vi "MaterialConvert.vi"(8 "Colors Cluster":T1 {"Material"."Shine" format="%.2f"}, 9 "Array":i32[](array[numeric]), 10 "Scene.Geometry.New Mesh":refnum<vi>, 11 "Scene.New Object":refnum<vi>) -> (2 "Scene.New Object 2":refnum<vi>, 3 "Scene.Geometry.New Mesh 2":refnum<vi>)   [LabVIEW 2020, in "NI_3D Picture Control.lvlib"]
uses:
  <vilib>/picture/3D Picture Control/NI_3D Picture Control.lvlib
  <vilib>/picture/3D Picture Control/Old 3D Toolkit.llb/SkinCluster.ctl
  <vilib>/picture/3D Picture Control/Old 3D Toolkit.llb/SkinType.ctl
  <vilib>/picture/3D Picture Control/Old 3D Toolkit.llb/Material.ctl
  <vilib>/picture/3D Picture Control/NI_Old 3D Toolkit.lvlib
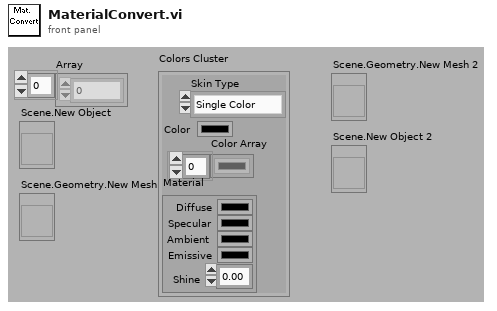
[diagram p1: front panel]
types:
  T1 = typedef "NI_3D Picture Control.lvlib/NI_Old 3D Toolkit.lvlib/SkinCluster.ctl" = cluster{"Skin Type":T2, "Color":u32, "Color Array":u32[], "Material":T3}
  T2 = typedef "NI_3D Picture Control.lvlib/NI_Old 3D Toolkit.lvlib/SkinType.ctl" = enum16{"Single Color", "Color per Vertex", "Material"}
  T3 = typedef "NI_3D Picture Control.lvlib/NI_Old 3D Toolkit.lvlib/Material.ctl" = cluster{"Diffuse":u32, "Specular":u32, "Ambient":u32, "Emissive":u32, "Shine":sgl}
  T4 = enum16{"Overall", "Per Primitive", "Per Vertex", "Binding Off"}
  T5 = enum16{"Inherit Material", "Use entire Material", "Ignore Ambient", "Ignore Diffuse", "Ignore Specular", "Ignore Emission", "Ignore Ambient and Diffuse"}
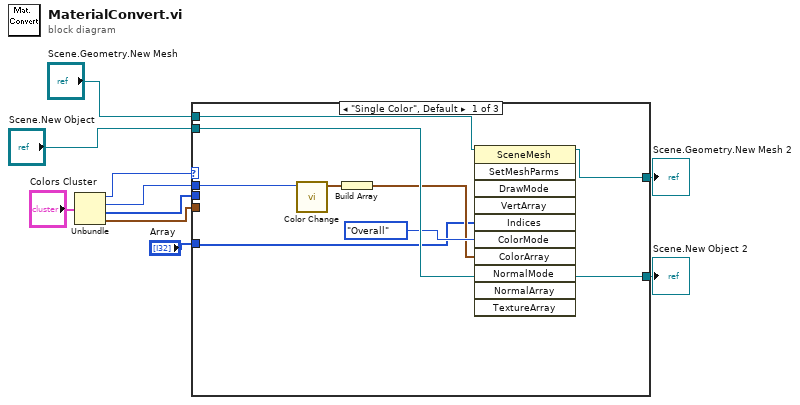
[diagram p0: block diagram]
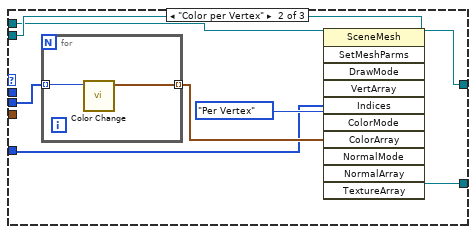
[diagram p2: hidden frame]
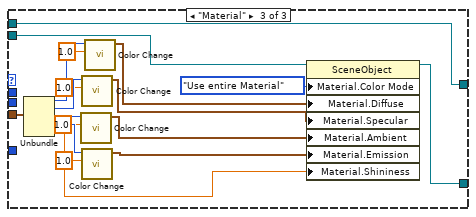
[diagram p3: hidden frame]
diagram:
  n1 = Unbundle("Colors Cluster") -> ("Skin Type"=w10:T2, "Color"=w7:u32, "Color Array"=w9:u32[], "Material"=w8:T3)
  n2 = case shown="\"Single Color\", Default" w10 {
    tunnel: w9 -> [_ w25 _]
    tunnel: w8 -> [_ _ w45]
    tunnel: "Scene.New Object" -> [w18 w24 w44]
    tunnel: w7 -> [w14 _ _]
    tunnel: [w18 w24 w39] -> w2
    tunnel: "Scene.Geometry.New Mesh" -> [w17 w23 w38]
    tunnel: "Array" -> [w11 w19 _]
    tunnel: [w16 w22 w38] -> w3
    frame "Single Color", Default {
      n3 = call <vilib>:"Color Change.vi"("Color"=w14) -> ("RGBA"=w13:cluster{"R":sgl, "G":sgl, "B":sgl, "A":sgl})  [unwired: 10 in]
      n4 = Build Array(w13) -> (w12:cluster{"R":sgl, "G":sgl, "B":sgl, "A":sgl}[])
      n5 = invoke class="SceneMesh" method="SetMeshParms"(reference=w17, "Indices"=w11, "ColorMode"=T4."Overall" ("Color Binding Mode"), "ColorArray"=w12) -> (reference out=w16:refnum<vi>)  [unwired: 7 in, 10 out]
    }
    frame "Color per Vertex" {
      n6 = for {
        tunnel: [w26] -> w20 mode=indexing
        tunnel: w25 -> [w27] mode=indexing
        n7 = call <vilib>:"Color Change.vi"("Color"=w27) -> ("RGBA"=w26:cluster{"R":sgl, "G":sgl, "B":sgl, "A":sgl})  [unwired: 10 in]
      }
      n8 = invoke class="SceneMesh" method="SetMeshParms"(reference=w23, "Indices"=w19, "ColorMode"=enum16{"Overall", "Per Primitive", "Per Vertex"}."Per Vertex" ("Color Binding Mode"), "ColorArray"=w20) -> (reference out=w22:refnum<vi>)  [unwired: 7 in, 10 out]
    }
    frame "Material" {
      n9 = Unbundle(w45) -> ("Diffuse"=w43:u32, "Specular"=w42:u32, "Ambient"=w41:u32, "Emissive"=w40:u32, "Shine"=w34:sgl)
      n10 = call <vilib>:"Color Change.vi"("Alpha"=1.0, "Color"=w41) -> ("RGBA"=w33:cluster{"R":sgl, "G":sgl, "B":sgl, "A":sgl})  [unwired: 9 in]
      n11 = call <vilib>:"Color Change.vi"("Alpha"=1.0, "Color"=w42) -> ("RGBA"=w35:cluster{"R":sgl, "G":sgl, "B":sgl, "A":sgl})  [unwired: 9 in]
      n12 = call <vilib>:"Color Change.vi"("Alpha"=1.0, "Color"=w40) -> ("RGBA"=w32:cluster{"R":sgl, "G":sgl, "B":sgl, "A":sgl})  [unwired: 9 in]
      n13 = call <vilib>:"Color Change.vi"("Alpha"=1.0, "Color"=w43) -> ("RGBA"=w36:cluster{"R":sgl, "G":sgl, "B":sgl, "A":sgl})  [unwired: 9 in]
      n14 = property class="SceneObject"(reference=w44, "Material.Color Mode"=T5."Use entire Material" ("Material:Color Mode"), "Material.Diffuse"=w36, "Material.Specular"=w35, "Material.Ambient"=w33, "Material.Emission"=w32, "Material.Shininess"=w34) -> (reference out=w39:refnum<vi>)  [unwired: 1 in, 1 out]
    }
  }
  "Scene.Geometry.New Mesh 2" <- w3
  "Scene.New Object 2" <- w2
